vi "Gaussian_Mixture_with_iris_data.vi"() -> ()   [LabVIEW 2020]
doc: "Using gaussian mixture to make clusters with the iris dataset."
uses:
  Model/Unsupervised/Mixture/GaussianMixture/Controls/gaussian_mixture_params.ctl
  4892a6b6-237d-49db-85c0-d0051253a407.vi
  Model/Unsupervised/Mixture/GaussianMixture/GaussianMixture.lvclass
  C:/Users/cipop/TDF Dropbox/2_Technologies de France/1 - Services et Etudes/PLAIY/2 - DEV/PLAIYLAB/code/Model/Model.lvclass
  C:/Users/cipop/TDF Dropbox/2_Technologies de France/1 - Services et Etudes/PLAIY/2 - DEV/PLAIYLAB/code/Model/Unsupervised/Mixture/Mixture.lvclass
  Model/Unsupervised/Mixture/GaussianMixture/GaussianMixture.vi
  <vilib>/Utility/file.llb/Application Directory.vi
  <vilib>/Platform/system.llb/System Exec.vi
panel:
  out "standard error":string
  out "error out":errorcluster
  out "XY Graph":T1(graph)
  in  "params":T2={"n_components"=3.0, "covariance_type"="full", "tol"=0.001, "reg_covar"=1e-06, "max_iter"=100.0, "n_init"=1.0, "init_params"="kmeans", "weights_init"={"weights_init_type"="None", "weights_init_list"=[]}, "means_init"={"means_init_type"="None", "means_init_list"=[]}, "precisions_init"={"precisions_init_type"="None", "precisions_init_list"=[]}, "random_state"=0.0, "warm_start"=FALSE, "verbose"=0.0, "verbose_interval"=10.0}
  out "X":dbl[][](array[numeric])
  out "y":string[][](array[string])
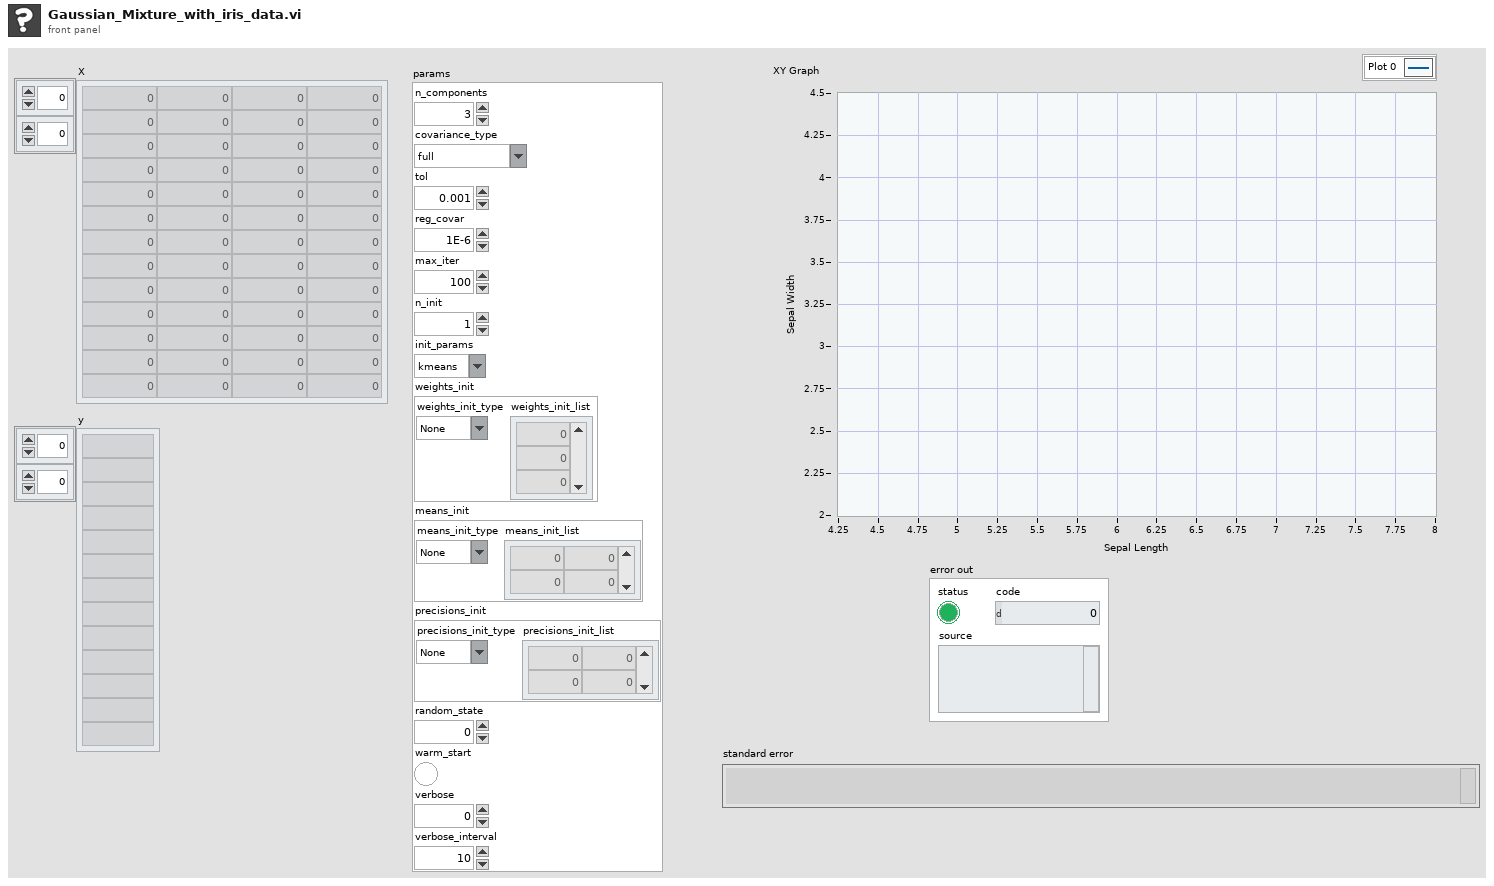
[diagram p1: front panel]
types:
  T1 = cluster{"XY Graph":cluster{"X":dbl, "Y":dbl}[]}[]
  T2 = typedef "gaussian_mixture_params.ctl" = cluster{"n_components":dbl, "covariance_type":string, "tol":dbl, "reg_covar":dbl, "max_iter":dbl, "n_init":dbl, "init_params":string, "weights_init":cluster{"weights_init_type":string, "weights_init_list":dbl[]}, "means_init":cluster{"means_init_type":string, "means_init_list":dbl[][]}, "precisions_init":cluster{"precisions_init_type":string, "precisions_init_list":dbl[][]}, "random_state":dbl, "warm_start":bool, "verbose":dbl, "verbose_interval":dbl}
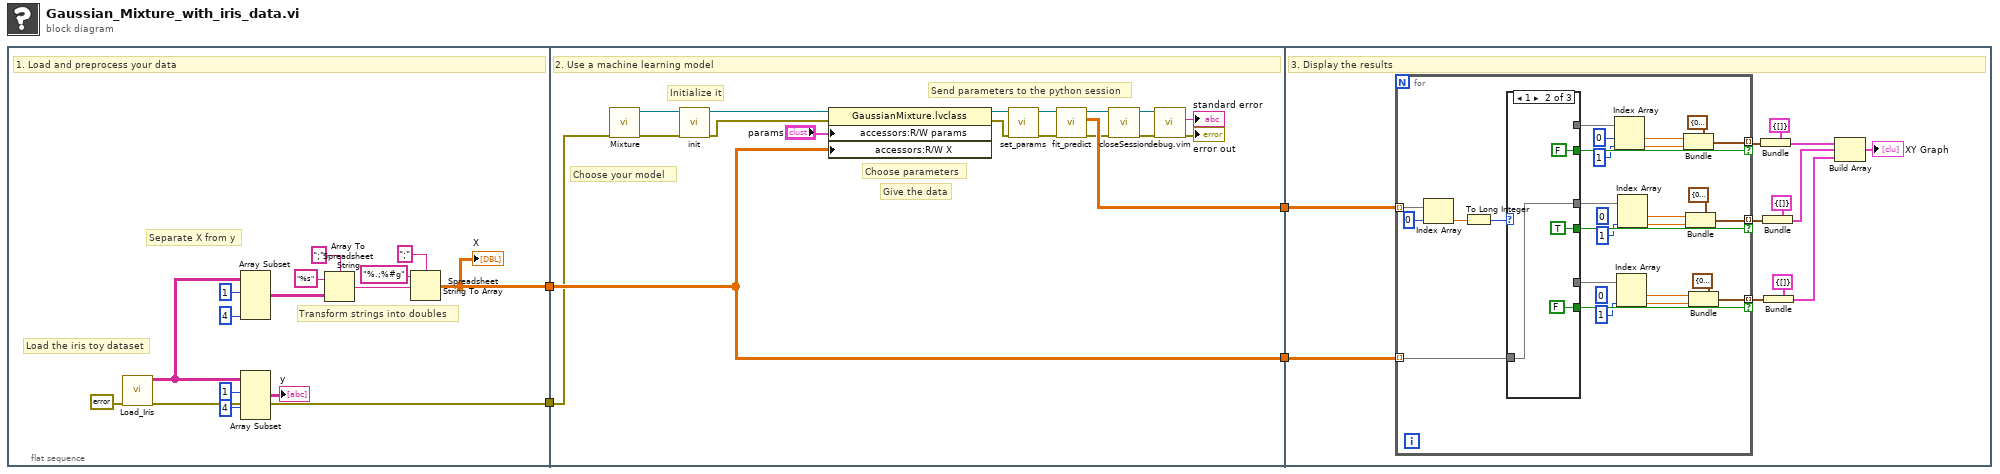
[diagram p0: block diagram]
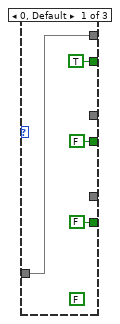
[diagram p2: hidden frame]
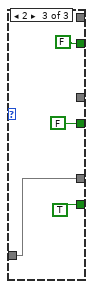
[diagram p3: hidden frame]
diagram:
  n1 = flat-sequence {
    tunnel: [w6] -> w4
    tunnel: [w5] -> w1
    tunnel: w4 -> [w28]
    tunnel: [w29] -> w3
    tunnel: [w28] -> w2
    tunnel: w1 -> [w22]
    tunnel: w3 -> [w48]
    tunnel: w2 -> [w49]
    frame #0 {
      # "Separate X from y"
      # "Transform strings into doubles"
      # "Load the iris toy dataset"
      # "1. Load and preprocess your data"
      n2 = call "Load_Iris.vi"("error in"=errorcluster {"status"=FALSE, "code"=0, "source"=""}) -> ("error out"=w5:errorcluster, "Tableau"=w14:string[][])  [unwired: 9 in]
      n3 = Array Subset(array=w14, index (row)=1 ("index"), length (col)=4 ("length")) -> (w12:string[][])  [unwired: 2 in]
      n4 = Array Subset(array=w14, index (row)=1 ("index"), index (col)=4 ("index")) -> (→"y":string[][])  [unwired: 2 in]
      n5 = Array To Spreadsheet String(delimiter (Tab)=";", array=w12, 3:"%s" ("format string")) -> (spreadsheet string=w7:string)
      n6 = Spreadsheet String To Array(delimiter (Tab)=";", format string="%.;%#g", spreadsheet string=w7) -> (array=w6:dbl[][])  [unwired: 1 in]
      "X" <- w6
    }
    frame #1 {
      # "Send parameters to the python session"
      # "Give the data"
      # "Choose parameters"
      # "Initialize it"
      # "Choose your model"
      # "2. Use a machine learning model"
      n7 = call-poly "Mixture.vi"("error in"=w22) -> ("error out"=w27:errorcluster, "out"=w34:refnum<class "GaussianMixture.lvclass">)  [unwired: 9 in]
      n8 = call-dynamic "init.vi"("error in (no error)"=w27, "Model en entrée"=w34) -> ("error out"=w36:errorcluster, "Model en sortie"=w35:refnum<class "GaussianMixture.lvclass">)  [unwired: 8 in]
      n9 = property class="GaussianMixture.lvclass"(reference=w35, error in=w36, "accessors:R/W params"="params", "accessors:R/W X"=w28) -> (reference out=w33:refnum<class "GaussianMixture.lvclass">, error out=w31:errorcluster)
      n10 = call-dynamic "set_params.vi"("error in (no error)"=w31, "GaussianMixture.lvclass 2"=w33) -> ("error out"=w30:errorcluster, "GaussianMixture.lvclass"=w32:refnum<class "GaussianMixture.lvclass">)  [unwired: 8 in]
      n11 = call-dynamic "fit_predict.vi"("error in (no error)"=w30, "Mixture.lvclass 2"=w32) -> ("error out"=w20:errorcluster, "C"=w29:dbl[][], "Mixture.lvclass"=w21:refnum<class "GaussianMixture.lvclass">)  [unwired: 7 in]
      n12 = call-dynamic "closeSession.vi"("error in"=w20, "Python en entrée"=w21) -> ("error out"=w25:errorcluster, "Python en sortie"=w26:refnum<class "GaussianMixture.lvclass">)  [unwired: 8 in]
      n13 = call "debug.vim"("error in (no error)"=w25, "Model.lvclass"=w26) -> ("error out"=→"error out":errorcluster, "standard error"=→"standard error":string)  [unwired: 7 in, 1 out]
    }
    frame #2 {
      # "3. Display the results"
      n14 = for {
        tunnel: w49 -> [w72] mode=indexing
        tunnel: w48 -> [w76] mode=indexing
        tunnel: [w52] -> w46 mode=indexing if=w71
        tunnel: [w51] -> w44 mode=indexing if=w70
        tunnel: [w50] -> w42 mode=indexing if=w69
        (unwired) 0 ("index")
        (unwired) 0 ("index")
        n15 = Index Array(array=w76, index=0) -> (element=w74:dbl)
        n16 = To Long Integer(number=w74) -> (32bit integer=w73:i32)
        n17 = case shown="1" w73 {
          tunnel: w72 -> [w80 w83 w86]
          tunnel: [w80 _ _] -> w67
          tunnel: [TRUE FALSE FALSE] -> w71
          tunnel: [_ w83 _] -> w61
          tunnel: [FALSE TRUE FALSE] -> w70
          tunnel: [_ _ w86] -> w62
          tunnel: [FALSE FALSE TRUE] -> w69
          frame 0, Default {
            (unwired) FALSE
          }
          frame 1 {
          }
          frame 2 {
          }
        }
        n18 = Index Array(array=w67, index #1=0 ("index"), index #2=1 ("index")) -> (element #1=w60:dbl, element #2=w59:dbl)
        n19 = Index Array(array=w62, index #2=1 ("index")) -> (element #1=w53:dbl, element #2=w54:dbl)  [unwired: 1 in]
        n20 = Index Array(array=w61, index #2=1 ("index")) -> (element #1=w56:dbl, element #2=w55:dbl)  [unwired: 1 in]
        n21 = Bundle(cluster=cluster{"X":dbl, "Y":dbl} {"X"=0.0, "Y"=0.0}, "X"=w60, "Y"=w59) -> (w52:cluster{"X":dbl, "Y":dbl})
        n22 = Bundle(cluster=cluster{"X":dbl, "Y":dbl} {"X"=0.0, "Y"=0.0}, "X"=w56, "Y"=w55) -> (w51:cluster{"X":dbl, "Y":dbl})
        n23 = Bundle(cluster=cluster{"X":dbl, "Y":dbl} {"X"=0.0, "Y"=0.0}, "X"=w53, "Y"=w54) -> (w50:cluster{"X":dbl, "Y":dbl})
      }
      n24 = Bundle(cluster=cluster{"XY Graph":cluster{"X":dbl, "Y":dbl}[]} {"XY Graph"=[]}, "XY Graph"=w46) -> (w41:cluster{"XY Graph":cluster{"X":dbl, "Y":dbl}[]})
      n25 = Bundle(cluster=cluster{"XY Graph":cluster{"X":dbl, "Y":dbl}[]} {"XY Graph"=[]}, "XY Graph"=w44) -> (w40:cluster{"XY Graph":cluster{"X":dbl, "Y":dbl}[]})
      n26 = Bundle(cluster=cluster{"XY Graph":cluster{"X":dbl, "Y":dbl}[]} {"XY Graph"=[]}, "XY Graph"=w42) -> (w39:cluster{"XY Graph":cluster{"X":dbl, "Y":dbl}[]})
      n27 = Build Array(w41, w40, w39) -> (→"XY Graph":T1)
    }
  }
